vi "Ctor.vi"(8 "error in (no error)":errorcluster, 11 "ByRef Base in":refnum<class "ByRef Base.lvclass">) -> (0 "error out":errorcluster, 3 "ByRef Base out":refnum<class "ByRef Base.lvclass">)   [LabVIEW 2012, in "ByRef Base.lvclass"]
uses:
  ByRef Base.lvclass
  Ref Data.ctl
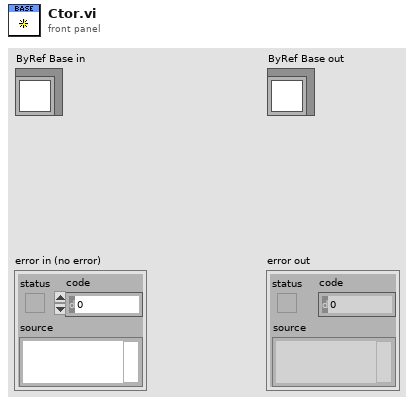
[diagram p1: front panel]
types:
  T1 = typedef "ByRef Base.lvclass/Ref Data.ctl" = cluster{"A":dbl, "B":dbl}
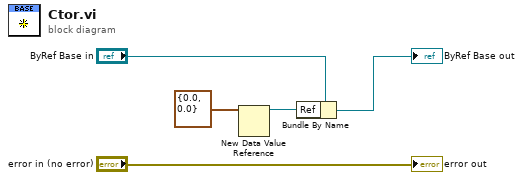
[diagram p0: block diagram]
diagram:
  n1 = New Data Value Reference(data value=T1 {"A"=0.0, "B"=0.0} ("Ref Data")) -> (data value reference=w1:refnum<data-value>)  [unwired: 1 in, 1 out]
  n2 = Bundle By Name(cluster="ByRef Base in", "Ref"=w1) -> (→"ByRef Base out":refnum<class "ByRef Base.lvclass">)
  "error out" <- "error in (no error)"
